vi "run_chatcompletion_core.vi"(0 "llm_ollama_chatmodels in":refnum<class "llm_ollama_chatmodels.lvclass">, 5 "Messages":refnum<class "abstract_message_base.lvclass">[](array[class]), 11 "error in (no error)":errorcluster) -> (4 "llm_ollama_chatmodels out":refnum<class "llm_ollama_chatmodels.lvclass">, 6 "Response":refnum<class "abstract_message_base.lvclass">, 15 "error out":errorcluster)   [LabVIEW 2020, in "llm_ollama_chatmodels.lvclass"]
uses:
  llm_ollama_chatmodels.lvclass
  abstract_message_base/abstract_message_base.lvclass
  message_text/message_text.lvclass
  D:/Personal/LabVIEW LLMs/src/models/abstract_message_base/abstract_message_base.lvclass
  message_text/message.ctl
  <vilib>/httpClient/POSTBuffer.vi
  <vilib>/httpClient/LabVIEWHTTPClient.lvlib
panel:
  out "body":string
  out "headers":string
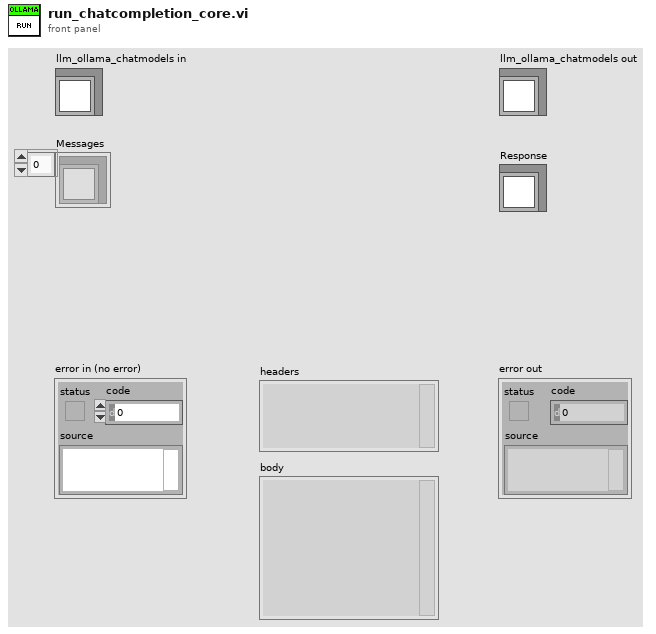
[diagram p1: front panel]
types:
  T1 = typedef "message_text.lvclass/message.ctl" = cluster{"role":string, "content":string[]}
  T2 = typedef "LabVIEWHTTPClient.lvlib/ClientHandle.ctl" = refnum<k1>
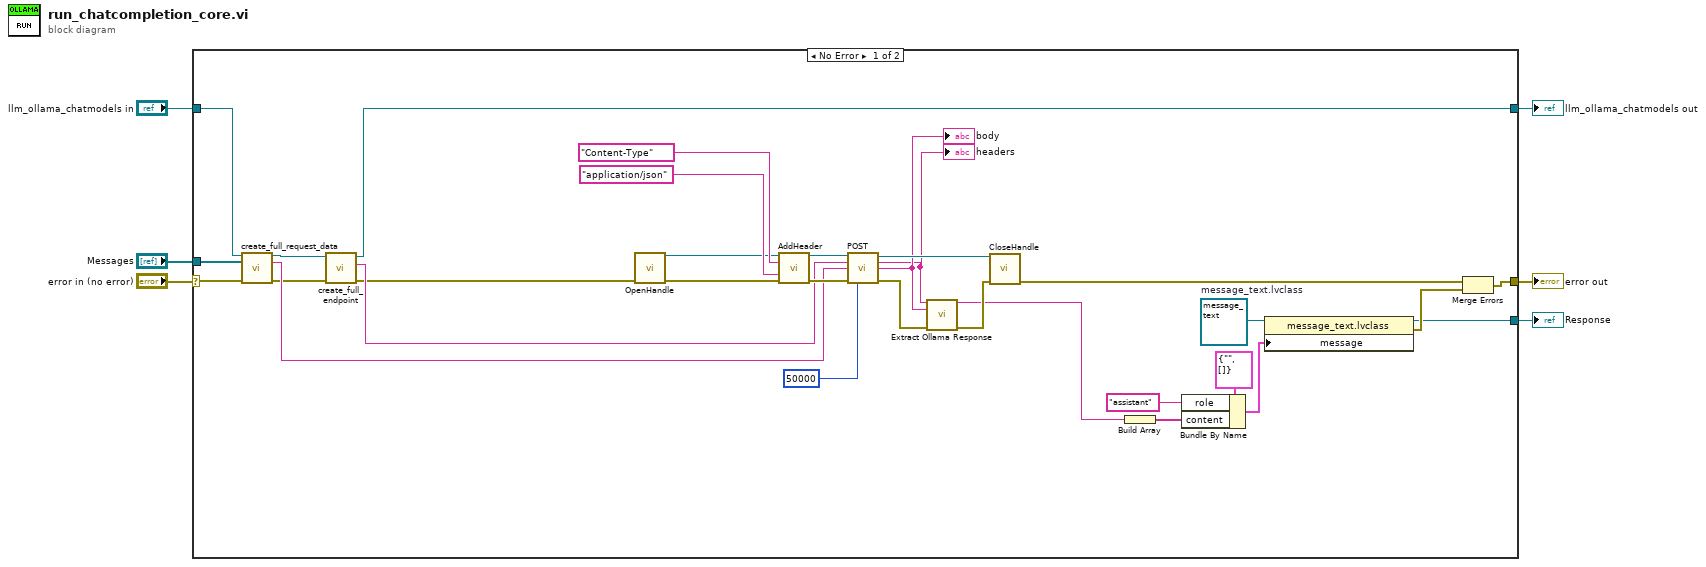
[diagram p0: block diagram]
diagram:
  n1 = case shown="No Error" "error in (no error)" {
    selector: "error in (no error)" -> [w22 w39]
    tunnel: [w25 w39] -> w5
    tunnel: "llm_ollama_chatmodels in" -> [w24 w38]
    tunnel: [w16 w38] -> w3
    tunnel: "Messages" -> [w23 _]
    tunnel: [w7 _] -> w1
    frame No Error {
      w14 = refnum<class "message_text.lvclass"> refnum  # message_text.lvclass
      n2 = call-dynamic "create_full_request_data.vi"("llm_ollama_chatmodels in"=w24, "Messages"=w23, "error in (no error)"=w22) -> ("llm_ollama_chatmodels out"=w20:refnum<class "llm_ollama_chatmodels.lvclass">, "Request Data"=w21:string, "error out"=w19:errorcluster)  [unwired: 10 in]
      n3 = call-dynamic "create_full_endpoint.vi"("error in (no error)"=w19, "llm_openai_chatmodels in"=w20) -> ("error out"=w17:errorcluster, "endpoint"=w18:string, "llm_openai_chatmodels out"=w16:refnum<class "llm_ollama_chatmodels.lvclass">)  [unwired: 7 in]
      n4 = call <vilib>:"OpenHandle.vi"("error in (no error)"=w17) -> ("client handle out"=w35:T2, "error out"=w33:errorcluster)  [unwired: 13 in]
      n5 = call <vilib>:"AddHeader.vi"("client handle"=w35, "header"="Content-Type", "value"="application/json", "error in (no error)"=w33) -> ("client handle out"=w34:T2, "error out"=w32:errorcluster)  [unwired: 10 in]
      n6 = call-poly <vilib>:"POST.vi"("client handle"=w34, "url"=w18, "buffer"=w21, "error in (no error)"=w32, "timeout (10000)"=50000) -> ("client handle out"=w30:T2, "headers"=w26:string, "body"=w27:string, "error out"=w29:errorcluster)  [unwired: 7 in]
      "headers" <- w26
      "body" <- w27
      n7 = call "Extract Ollama Response.vi"("headers"=w26, "body"=w27, "error in"=w29) -> ("value"=w9:string, "error out"=w28:errorcluster)  [unwired: 11 in]
      n8 = call <vilib>:"CloseHandle.vi"("client handle"=w30, "error in (no error)"=w28) -> ("error out"=w31:errorcluster)  [unwired: 13 in]
      n9 = Build Array(w9) -> (w11:string[])
      n10 = Bundle By Name(cluster=T1 {"role"="", "content"=[]} ("message"), "role"="assistant", "content"=w11) -> (w10:T1)
      n11 = property class="message_text.lvclass"(reference=w14, "message"=w10) -> (reference out=w7:refnum<class "message_text.lvclass">, error out=w8:errorcluster)  [unwired: 1 in]
      n12 = Merge Errors(w31, w8) -> (w25:errorcluster)
    }
    frame Error {
    }
  }
  "error out" <- w5
  "llm_ollama_chatmodels out" <- w3
  "Response" <- w1
